vi "Cubodecolores2.vi"() -> ()   [LabVIEW 2016]
panel:
  in  "Horizontal Pointer Slide":dbl(slide) scale=0.0..255.0
  out "new picture":picture
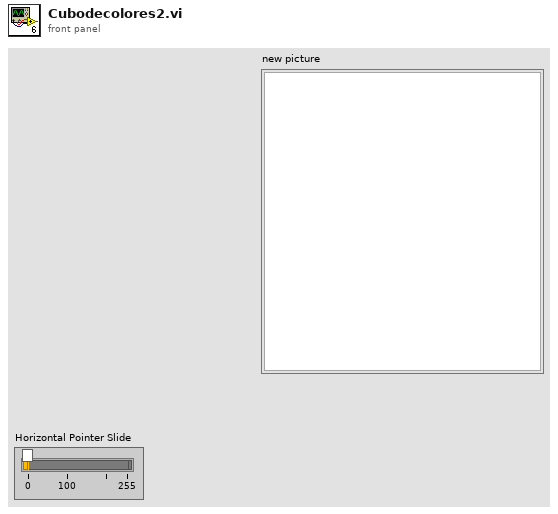
[diagram p1: front panel]
types:
  T1 = typedef "imagedata.ctl" = cluster{"image type":i32, "image depth":i32, "image":u8[], "mask":u8[], "colors":u32[], "Rectangle":cluster{"left":i16, "top":i16, "right":i16, "bottom":i16}}
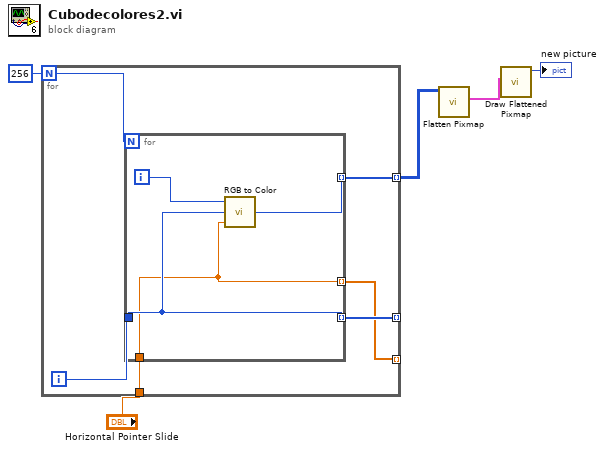
[diagram p0: block diagram]
diagram:
  n1 = for {
    N: 256 -> [w11]
    tunnel: [w9] -> w4 mode=indexing
    tunnel: [w8] -> _ mode=indexing
    tunnel: [w7] -> _ mode=indexing
    tunnel: "Horizontal Pointer Slide" -> [w6]
    i -> [w10]
    n2 = for {
      N: w11 -> [_]
      tunnel: [w13] -> w9 mode=indexing
      tunnel: w10 -> [w14]
      tunnel: [w14] -> w8 mode=indexing
      tunnel: [w12] -> w7 mode=indexing
      tunnel: w6 -> [w12]
      i -> [w15]
      n3 = call <vilib>:"RGB to Color.vi"("B"=w12, "G"=w14, "R"=w15) -> ("Color"=w13:u32)
    }
  }
  n4 = call <vilib>:"Flatten Pixmap.vi"("24-bit pixmap"=w4) -> ("image data"=w3:T1)  [unwired: 10 in]
  n5 = call <vilib>:"Draw Flattened Pixmap.vi"("image data"=w3) -> ("new picture"=→"new picture":picture)  [unwired: 8 in]
